vi "Get Modules List.vi"(0 "SLSC Remote in":refnum<class "SLSC Remote.lvclass">, 11 "error in (no error)":errorcluster) -> (4 "SLSC Remote out":refnum<class "SLSC Remote.lvclass">, 8 "Sys.Modules":refnum<k21>[](array[refnum]), 15 "error out":errorcluster)   [LabVIEW 2016, in "SLSC Interfaces.lvlib" / "SLSC Remote.lvclass"]
uses:
  SLSC Remote.lvclass
  C:/Users/tblair/Documents/Git Projects/SLSC-Interface/Source/SLSC Interface Class/SLSC Interface.lvclass
  <vilib>/National Instruments/JSON Support for LabVIEW/JSON Data Classes/JSON Object/JSON Object.lvclass
  C:/Program Files (x86)/National Instruments/LabVIEW 2016/vi.lib/National Instruments/JSON Support for LabVIEW/JSON Data Classes/JSON Datatype/JSON Datatype.lvclass
  <vilib>/National Instruments/JSON Support for LabVIEW/JSON Data Classes/JSON Object/New JSON Object (Empty).vi
  <vilib>/National Instruments/JSON Support for LabVIEW/JSON Data Classes/JSON Object/Insert Key Value Pair (Single String).vi
  <vilib>/NI/NI JSONRPC Server Framework/Classes/Server/Format Client Request (Auto-Increment).vi
  <vilib>/httpClient/POSTBuffer.vi
  <vilib>/National Instruments/JSON Support for LabVIEW/JSON Data Classes/JSON Datatype/To More Specific Type (Object).vi
  <vilib>/National Instruments/JSON Support for LabVIEW/JSON Data Classes/JSON Object/Get Value (Array).vi
  <vilib>/National Instruments/JSON Support for LabVIEW/JSON Data Classes/JSON Array/Index Array (String Value).vi
  <vilib>/NI/NI JSONRPC Server Framework/Classes/Server/JSONRPC Server.lvclass
  <vilib>/httpClient/LabVIEWHTTPClient.lvlib
  <vilib>/National Instruments/JSON Support for LabVIEW/JSON Data Classes/JSON Datatype/JSON Datatype.lvclass
  <vilib>/National Instruments/JSON Support for LabVIEW/JSON Data Classes/JSON Array/JSON Array.lvclass
  C:/Program Files (x86)/National Instruments/LabVIEW 2016/vi.lib/National Instruments/JSON Support for LabVIEW/JSON Data Classes/JSON Structured Type/JSON Structured Type.lvclass
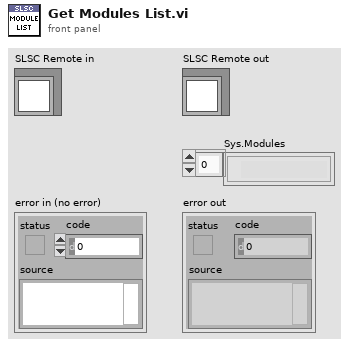
[diagram p1: front panel]
types:
  T1 = typedef "LabVIEWHTTPClient.lvlib/ClientHandle.ctl" = refnum<k1>
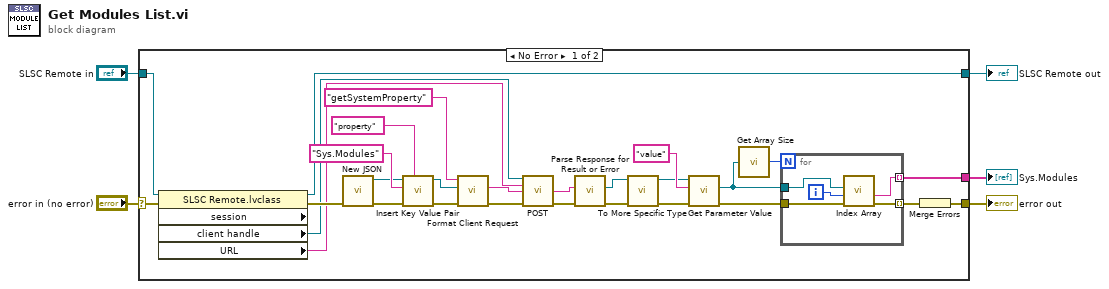
[diagram p0: block diagram]
diagram:
  n1 = case shown="No Error" "error in (no error)" {
    selector: "error in (no error)" -> [w31 w39]
    tunnel: "SLSC Remote in" -> [w33 w40]
    tunnel: [w32 w40] -> w3
    tunnel: [w9 w39] -> w1
    tunnel: [w10 _] -> w2
    frame No Error {
      n2 = property class="SLSC Remote.lvclass" props=["session", "client handle", "URL"](reference=w33, error in=w31) -> (reference out=w32:refnum<class "SLSC Remote.lvclass">, error out=w30:errorcluster, "client handle"=w26:T1, "URL"=w25:string)  [unwired: 1 out]
      n3 = call-poly <vilib>:"New JSON.vi"("error in (no error)"=w30) -> ("error out"=w29:errorcluster, "JSON Object out"=w6:refnum<class "JSON Object.lvclass">)  [unwired: 9 in]
      n4 = call-poly <vilib>:"Insert Key Value Pair.vi"("key"="property" ("Name"), "error in (no error)"=w29, "value"="Sys.Modules" ("String"), "JSON Object in"=w6) -> ("error out"=w20:errorcluster, "JSON Object out"=w21:refnum<class "JSON Object.lvclass">)  [unwired: 5 in, 1 out]
      n5 = call-poly <vilib>:"Format Client Request.vi"("error in (no error)"=w20, "JSON in"=w21, "method"="getSystemProperty") -> ("error out"=w24:errorcluster, "Request String"=w27:string)  [unwired: 7 in]
      n6 = call-poly <vilib>:"POST.vi"("client handle"=w26, "url"=w25, "buffer"=w27, "error in (no error)"=w24) -> ("body"=w23:string, "error out"=w22:errorcluster)  [unwired: 8 in, 2 out]
      n7 = call <vilib>:"Parse Response for Result or Error.vi"("error in"=w22, "Response String In"=w23) -> ("error out"=w11:errorcluster, "JSON out"=w12:refnum<class "JSON Datatype.lvclass">)  [unwired: 7 in, 1 out]
      n8 = call-poly <vilib>:"To More Specific Type.vi"("error in (no error)"=w11, "JSON Datatype in"=w12) -> ("error out"=w18:errorcluster, "JSON Datatype out"=w17:refnum<class "JSON Object.lvclass">)  [unwired: 8 in]
      n9 = call-poly <vilib>:"Get Parameter Value.vi"("error in (no error)"=w18, "key"="value" ("Parameter Name"), "JSON Object in"=w17) -> ("error out"=w14:errorcluster, "value"=w15:refnum<class "JSON Array.lvclass">)  [unwired: 6 in, 1 out]
      n10 = call <vilib>:"Get Array Size.vi"("JSON Array in"=w15) -> ("size(s)"=w16:i32)
      n11 = for {
        N: w16 -> [_]
        tunnel: w15 -> [w37]
        tunnel: w14 -> [w36]
        tunnel: [w35] -> w13 mode=indexing
        tunnel: [w34] -> w10 mode=indexing
        i -> [w38]
        n12 = call-poly <vilib>:"Index Array.vi"("error in (no error)"=w36, "index"=w38, "JSON Array in"=w37) -> ("error out"=w35:errorcluster, "String"=w34:string)  [unwired: 7 in]
      }
      n13 = Merge Errors(w13) -> (w9:errorcluster)
    }
    frame Error {
    }
  }
  "error out" <- w1
  "SLSC Remote out" <- w3
  "Sys.Modules" <- w2
